vi "Typecast Value and Format to String.vi"(7 "format string":string, 8 "error in (no error)":errorcluster, 9 "Data Type":T1, 10 "Endianess":T2, 11 "byte array":u8[](array[numeric])) -> (0 "error out":errorcluster, 3 "Formatted string":string)   [LabVIEW 2021, in "Ring Buffer Strict Accessor.lvlib"]
uses:
  Ring Buffer Strict Accessor.lvlib
  Endianess.ctl
  DataType.ctl
  938b3e23-a312-4fbb-a8e5-40c5536b82af.vi
  cd911914-4f53-475c-9ce4-21d55b2f7dc8.vi
  de9861ff-63fa-4a4b-9126-987b7a8373d8.vi
  604e4ae3-9afc-4fb6-82b9-5d0a2bb30445.vi
  de8e4c4f-05b4-4262-9144-9cc967ac4e1d.vi
  35635685-acbf-486d-94f5-1f6649101f82.vi
  a513d100-0ba6-48e1-9ead-670cf902c812.vi
  5110f586-3a5c-4a1a-968f-0589393c07d6.vi
  5e9e855d-e6a5-4302-a4d0-c6eb76946128.vi
  9717dc24-18f4-4b0e-8a3f-9d91d226a93e.vi
  c812d856-3863-456b-9754-0fe388b7ccba.vi
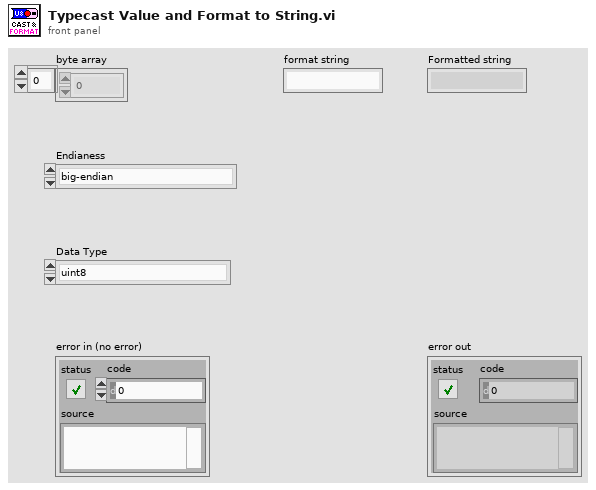
[diagram p1: front panel]
types:
  T1 = typedef "Ring Buffer Strict Accessor.lvlib/DataType.ctl" = enum16{"uint8", "uint16", "uint32", "uint64", "int8", "int16", "int32", "int64", "float", "double", "extended"}
  T2 = typedef "Ring Buffer Strict Accessor.lvlib/Endianess.ctl" = enum16{"big-endian", "little-endian"}
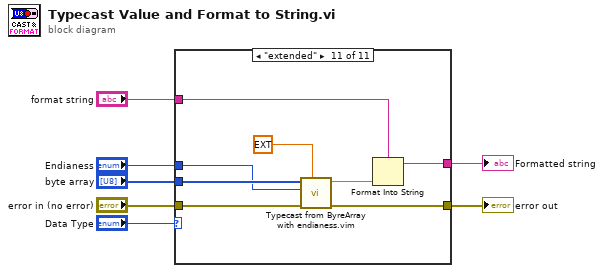
[diagram p0: block diagram]
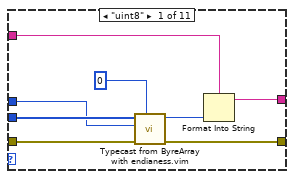
[diagram p2: hidden frame]
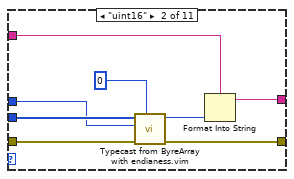
[diagram p3: hidden frame]
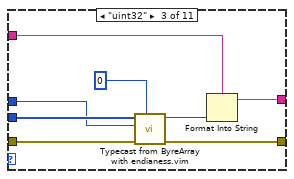
[diagram p4: hidden frame]
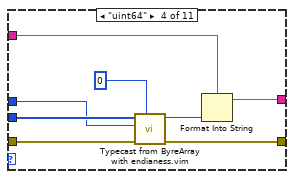
[diagram p5: hidden frame]
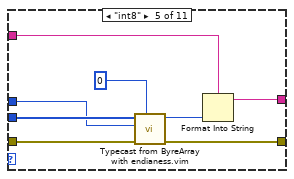
[diagram p6: hidden frame]
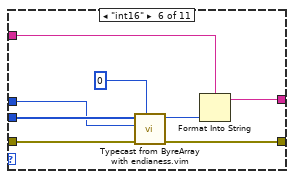
[diagram p7: hidden frame]
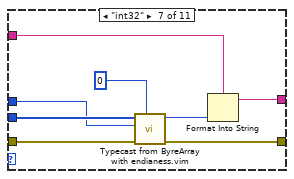
[diagram p8: hidden frame]
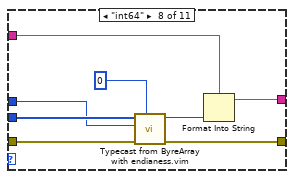
[diagram p9: hidden frame]
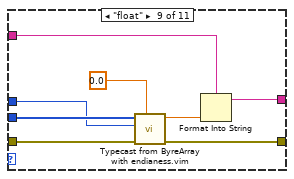
[diagram p10: hidden frame]
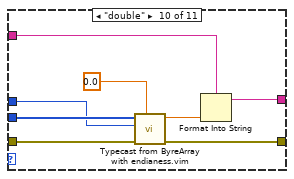
[diagram p11: hidden frame]
diagram:
  n1 = case shown="\"extended\"" "Data Type" {
    tunnel: "byte array" -> [w14 w22 w30 w38 w46 w54 w62 w70 w78 w87 w94]
    tunnel: "Endianess" -> [w13 w21 w29 w37 w45 w53 w61 w69 w77 w86 w93]
    tunnel: "format string" -> [w11 w19 w27 w35 w43 w51 w59 w67 w75 w83 w91]
    tunnel: [w10 w18 w26 w34 w42 w50 w58 w66 w74 w82 w90] -> w3
    tunnel: "error in (no error)" -> [w9 w17 w25 w33 w41 w49 w57 w65 w73 w81 w89]
    tunnel: [w8 w16 w24 w32 w40 w48 w56 w64 w72 w80 w88] -> w1
    frame "uint8" {
      n2 = call "Typecast from ByreArray with endianess.vim"("data type"=u8 0, "error in (no error)"=w9, "Endianess"=w13, "byte array"=w14) -> ("error out"=w8:errorcluster, "data"=w12:u8)  [unwired: 6 in]
      n3 = Format Into String(format string=w11, w12) -> (resulting string=w10:string)  [unwired: 2 in, 1 out]
    }
    frame "uint16" {
      n4 = call "Typecast from ByreArray with endianess.vim"("data type"=u16 0, "error in (no error)"=w17, "Endianess"=w21, "byte array"=w22) -> ("error out"=w16:errorcluster, "data"=w20:u16)  [unwired: 6 in]
      n5 = Format Into String(format string=w19, w20) -> (resulting string=w18:string)  [unwired: 2 in, 1 out]
    }
    frame "uint32" {
      n6 = call "Typecast from ByreArray with endianess.vim"("data type"=u32 0, "error in (no error)"=w25, "Endianess"=w29, "byte array"=w30) -> ("error out"=w24:errorcluster, "data"=w28:u32)  [unwired: 6 in]
      n7 = Format Into String(format string=w27, w28) -> (resulting string=w26:string)  [unwired: 2 in, 1 out]
    }
    frame "uint64" {
      n8 = call "Typecast from ByreArray with endianess.vim"("data type"=u64 0, "error in (no error)"=w33, "Endianess"=w37, "byte array"=w38) -> ("error out"=w32:errorcluster, "data"=w36:u64)  [unwired: 6 in]
      n9 = Format Into String(format string=w35, w36) -> (resulting string=w34:string)  [unwired: 2 in, 1 out]
    }
    frame "int8" {
      n10 = call "Typecast from ByreArray with endianess.vim"("data type"=i8 0, "error in (no error)"=w41, "Endianess"=w45, "byte array"=w46) -> ("error out"=w40:errorcluster, "data"=w44:i8)  [unwired: 6 in]
      n11 = Format Into String(format string=w43, w44) -> (resulting string=w42:string)  [unwired: 2 in, 1 out]
    }
    frame "int16" {
      n12 = call "Typecast from ByreArray with endianess.vim"("data type"=i16 0, "error in (no error)"=w49, "Endianess"=w53, "byte array"=w54) -> ("error out"=w48:errorcluster, "data"=w52:i16)  [unwired: 6 in]
      n13 = Format Into String(format string=w51, w52) -> (resulting string=w50:string)  [unwired: 2 in, 1 out]
    }
    frame "int32" {
      n14 = call "Typecast from ByreArray with endianess.vim"("data type"=0, "error in (no error)"=w57, "Endianess"=w61, "byte array"=w62) -> ("error out"=w56:errorcluster, "data"=w60:i32)  [unwired: 6 in]
      n15 = Format Into String(format string=w59, w60) -> (resulting string=w58:string)  [unwired: 2 in, 1 out]
    }
    frame "int64" {
      n16 = call "Typecast from ByreArray with endianess.vim"("data type"=i64 0, "error in (no error)"=w65, "Endianess"=w69, "byte array"=w70) -> ("error out"=w64:errorcluster, "data"=w68:i64)  [unwired: 6 in]
      n17 = Format Into String(format string=w67, w68) -> (resulting string=w66:string)  [unwired: 2 in, 1 out]
    }
    frame "float" {
      n18 = call "Typecast from ByreArray with endianess.vim"("data type"=sgl 0.0, "error in (no error)"=w73, "Endianess"=w77, "byte array"=w78) -> ("error out"=w72:errorcluster, "data"=w76:sgl)  [unwired: 6 in]
      n19 = Format Into String(format string=w75, w76) -> (resulting string=w74:string)  [unwired: 2 in, 1 out]
    }
    frame "double" {
      n20 = call "Typecast from ByreArray with endianess.vim"("data type"=0.0 ("Numeric"), "error in (no error)"=w81, "Endianess"=w86, "byte array"=w87) -> ("error out"=w80:errorcluster, "data"=w84:dbl)  [unwired: 6 in]
      n21 = Format Into String(format string=w83, w84) -> (resulting string=w82:string)  [unwired: 2 in, 1 out]
    }
    frame "extended" {
      n22 = call "Typecast from ByreArray with endianess.vim"("data type"=ext 0.0, "error in (no error)"=w89, "Endianess"=w93, "byte array"=w94) -> ("error out"=w88:errorcluster, "data"=w92:ext)  [unwired: 6 in]
      n23 = Format Into String(format string=w91, w92) -> (resulting string=w90:string)  [unwired: 2 in, 1 out]
    }
  }
  "Formatted string" <- w3
  "error out" <- w1
